vi "saturate.vi"(9 "Lower limit":dbl, 10 "In":dbl, 11 "Upper Limit":dbl) -> (3 "Out":dbl)   [LabVIEW 2018]
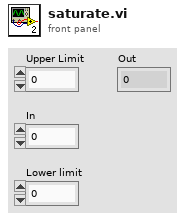
[diagram p1: front panel]
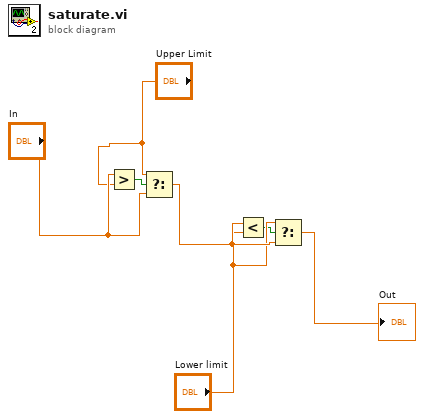
[diagram p0: block diagram]
diagram:
  n1 = Greater?(x="In", y="Upper Limit") -> (0:w1:bool)
  n2 = Select(t="Upper Limit", s=w1, f="In") -> (s? t:f=w6:dbl)
  n3 = Less?(x=w6, y="Lower limit") -> (x < y?=w4:bool)
  n4 = Select(t="Lower limit", s=w4, f=w6) -> (s? t:f=→"Out":dbl)
